vi "Server Connection Loop.vi"(8 "error in (no error)":errorcluster, 11 "TCPMessaging in":refnum<class "TCPMessaging.lvclass">) -> (0 "error out":errorcluster)   [LabVIEW 2020, in "Vecto.lvlib" / "TCPMessaging.lvclass"]
doc: "Listens for new incoming connections and spawns async client loops. The async client loops handle the handshake with the client app."
uses:
  TCPMessaging.lvclass
  TCPMessaging.lvclass/TCPMessaging.ctl
  Event Level.ctl
  EventLoggingService/EventLoggingService.lvclass/EventLoggingService.ctl
  <vilib>/Utility/error.llb/Error Cluster From Error Code.vi
  EventLogHandler/EventLogHandler.lvclass
  EventLoggingService/EventLoggingService.lvclass
  Vecto.lvlib
  IP Resolver/IP Resolver.lvclass
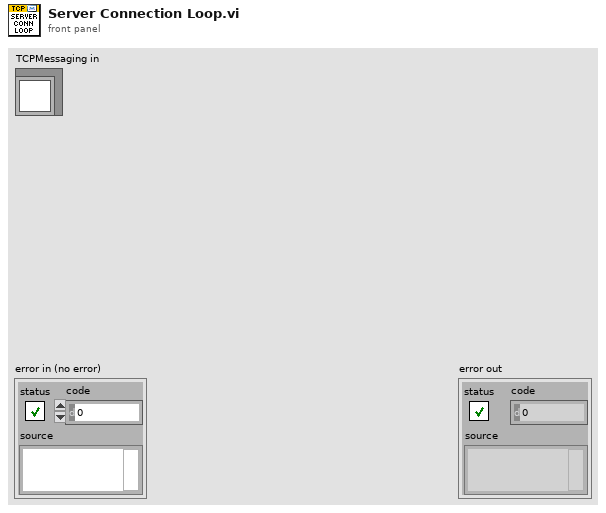
[diagram p1: front panel]
types:
  T1 = typedef "Vecto.lvlib/Event Level.ctl" = enum16{"Debug", "Info", "Warning", "Error"}
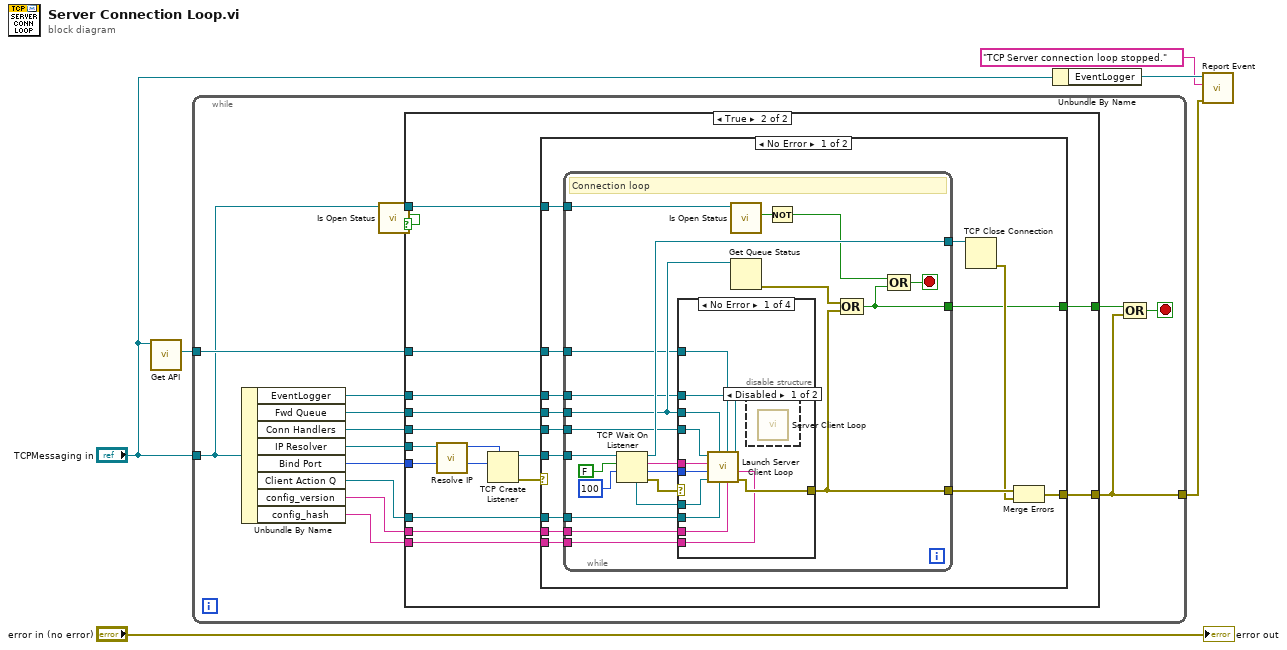
[diagram p0: block diagram]
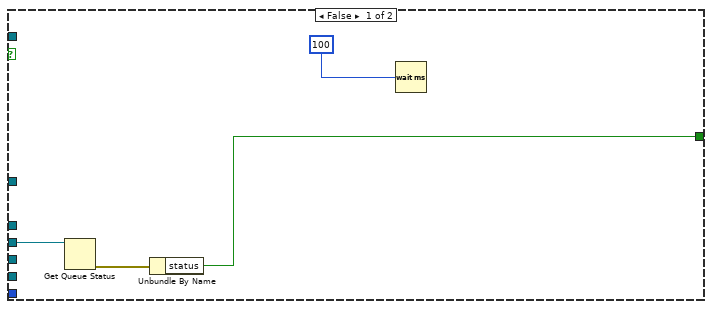
[diagram p2: hidden frame]
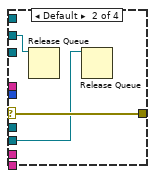
[diagram p4: hidden frame]
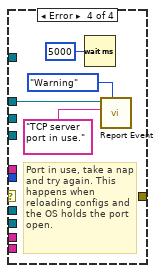
[diagram p6: hidden frame]
diagram:
  n1 = call "Get API.vi"("TCPMessaging in"="TCPMessaging in") -> ("TCP Messaging API"=w5:refnum<class "TCPMessageAPI.lvclass">)  [unwired: 8 in, 2 out]
  n2 = while {
    tunnel: "TCPMessaging in" -> [w11]
    tunnel: w5 -> [w16]
    tunnel: [w9] -> w1
    stop <- w8 stop-if-true
    n3 = Unbundle By Name(w11) -> ("EventLogger"=w14:refnum<class "EventLoggingService.lvclass">, "Fwd Queue"=w20:refnum<queue>, "Conn Handlers"=w15:refnum<queue>, "IP Resolver"=w7:refnum<class "IP Resolver.lvclass">, "Bind Port"=w21:u16, "Client Action Q"=w19:refnum<queue>, "config_version"=w13:string, "config_hash"=w12:string)
    n4 = call "Is Open Status.vi"("TCPMessaging in"=w11) -> ("Open"=w17:bool, "TCPMessaging out"=w18:refnum<class "TCPMessaging.lvclass">)  [unwired: 8 in, 1 out]
    n5 = case shown="True" w17 {
      tunnel: w21 -> [_ w40]
      tunnel: w20 -> [w24 w38]
      tunnel: w19 -> [_ w37]
      tunnel: w18 -> [_ w36]
      tunnel: [_ w30] -> w9
      tunnel: w16 -> [_ w35]
      tunnel: w15 -> [_ w34]
      tunnel: w14 -> [_ w33]
      tunnel: w13 -> [_ w32]
      tunnel: w12 -> [_ w31]
      tunnel: [w22 w29] -> w10
      tunnel: w7 -> [_ w27]
      frame False {
        n6 = Get Queue Status(queue=w24) -> (error out=w23:errorcluster)  [unwired: 2 in, 7 out]
        n7 = Unbundle By Name(w23) -> ("status"=w22:bool)
        n8 = Wait (ms)(milliseconds to wait=u32 100) -> ()  [unwired: 1 out]
      }
      frame True {
        n9 = call "Resolve IP.vi"("IP Resolver in"=w27) -> ("U32 Address"=w26:u32)  [unwired: 9 in, 1 out]
        n10 = TCP Create Listener(7:w26, 10:w40) -> (0:w28:errorcluster, 3:w39:refnum<k5>)  [unwired: 3 in, 1 out]
        n11 = case shown="No Error" w28 {
          selector: w28 -> [_ w95]
          tunnel: w39 -> [w54 _]
          tunnel: w38 -> [w53 _]
          tunnel: w37 -> [w52 _]
          tunnel: w36 -> [w51 _]
          tunnel: w35 -> [w48 _]
          tunnel: w34 -> [w47 _]
          tunnel: w33 -> [w46 _]
          tunnel: w32 -> [w45 _]
          tunnel: w31 -> [w44 _]
          tunnel: [w43 w95] -> w30
          tunnel: [w41 _] -> w29
          frame No Error {
            n12 = while {
              tunnel: w54 -> [w73]
              tunnel: w53 -> [w63]
              tunnel: w52 -> [w69]
              tunnel: w51 -> [w67]
              tunnel: [w65] -> w50
              tunnel: [w57] -> w49
              tunnel: w48 -> [w62]
              tunnel: w47 -> [w61]
              tunnel: w46 -> [w60]
              tunnel: w45 -> [w59]
              tunnel: w44 -> [w58]
              tunnel: [w55] -> w41
              stop <- w68 stop-if-true
              # "Connection loop"
              n13 = TCP Wait On Listener(9:100 ("timeout ms (wait forever: -1)"), 10:FALSE ("resolve remote address (T)"), 11:w73) -> (0:w74:errorcluster, 1:w72:u16, 2:w71:string, 3:w65:refnum<k5>, 4:w70:refnum<k5>)  [unwired: 1 in]
              n14 = case shown="No Error" w74 {
                selector: w74 -> [_ w90 _ _]
                tunnel: w72 -> [w86 _ _ _]
                tunnel: w71 -> [w87 _ _ _]
                tunnel: w70 -> [w85 _ _ _]
                tunnel: w63 -> [w83 w88 _ _]
                tunnel: w69 -> [w84 w89 _ _]
                tunnel: [w82 w90 _ _] -> w57
                tunnel: w62 -> [w81 _ _ _]
                tunnel: w61 -> [w80 _ _ _]
                tunnel: w60 -> [w79 _ _ w93]
                tunnel: w59 -> [w78 _ _ _]
                tunnel: w58 -> [w77 _ _ _]
                frame No Error {
                  n15 = call "Launch Server Client Loop.vi"("Local Hash"=w77, "Event Logging"=w79, "Local Version"=w78, "TCPMessageAPI"=w81, "Client Action Q"=w84, "Fwd Queue"=w83, "TCP Client"=w85, "Remote Port"=w86, "Remote Address"=w87, "Conn Handlers"=w80) -> ("error out"=w82:errorcluster)  [unwired: 1 in]
                  n16 = disable-structure shown="Disabled" {
                    frame Disabled {
                      n17 = call "Server Client Loop.vi"() -> ()  [unwired: 12 in]
                    }
                    frame Enabled {
                    }
                  }
                }
                frame Default {
                  n18 = Release Queue(queue=w88) -> ()  [unwired: 2 in, 3 out]
                  n19 = Release Queue(queue=w89) -> ()  [unwired: 2 in, 3 out]
                }
                frame Error {
                }
                frame Error {
                  # "Port in use, take a nap and try again. This happens when reloading configs and the OS holds the port open."
                  n20 = Wait (ms)(milliseconds to wait=u32 5000) -> ()  [unwired: 1 out]
                  n21 = call "Report Event.vi"("Event Level (Info)"=Event_Level."Warning", "Message"="TCP server port in use.", "EventLoggingService in"=w93) -> ()  [unwired: 7 in, 2 out]
                }
              }
              n22 = call "Is Open Status.vi"("TCPMessaging in"=w67) -> ("Open"=w66:bool)  [unwired: 8 in, 2 out]
              n23 = Get Queue Status(queue=w63) -> (error out=w56:errorcluster)  [unwired: 2 in, 7 out]
              n24 = Not(x=w66) -> (.not. x?=w64:bool)
              n25 = Compound Arithmetic op=OR(w56, w57) -> (w55:bool)
              n26 = Compound Arithmetic op=OR(w64, w55) -> (w68:bool)
            }
            n27 = TCP Close Connection(connection ID=w50) -> (error out=w42:errorcluster)  [unwired: 2 in, 1 out]
            n28 = Merge Errors(w49, w42) -> (w43:errorcluster)
          }
          frame Error {
          }
        }
      }
    }
    n29 = Compound Arithmetic op=OR(w10, w9) -> (w8:bool)
  }
  n30 = Unbundle By Name("TCPMessaging in") -> ("EventLogger"=w3:refnum<class "EventLoggingService.lvclass">)
  n31 = call "Report Event.vi"("error in (no error)"=w1, "Message"="TCP Server connection loop stopped.", "EventLoggingService in"=w3) -> ()  [unwired: 7 in, 2 out]
  "error out" <- "error in (no error)"
